vi "LINC Initialize.vi"(4 "override? registration":bool, 6 "configuration":T4={"header"=enum."STANDARD", "little endian (F)"=FALSE, "always write config (F)"=FALSE, "record commands (F)"=FALSE, "root COSMOS path (\"\")"=path "", "cmd record path (\"\")"=path "", "cmd interrupt (CMD)"="CMD", "tlm interrupt (TLM)"="TLM", "error interrupt (ERROR)"="ERROR", "default string bytes (50)"=50, "default array elements (50)"=50, "cmd length_bitoffset"=0, "cmd length_bitsize"=0, "cmd length_value_offset"=0, "tlm length_bitoffset"=0, "tlm length_bitsize"=0, "tlm length_value_offset"=0, "cmd GUID_bitoffset"=0, "tlm GUID_bitoffset"=0}, 7 "client session (F)":bool, 8 "error in (no error)":errorcluster, 9 "server name (\"\")":string, 10 "target name":string="APP", 11 "application queue":refnum<queue>) -> (0 "error out":errorcluster, 3 "LINC session":refnum<class "LINC.lvclass">)   [LabVIEW 2018, in "STEPkgDriver_LINC.lvlib" / "LINC.lvclass"]
uses:
  LINC.lvclass
  STEPkgDriver_LINC.lvlib
  LINC Global Mode.ctl
  LINC Global Session Mode.ctl
  LINC Global Config Mode.ctl
  LINC CCSDS Callback.vi
  LINC Config.ctl
  LINC Standard Callback.vi
  LINC Global Handshake Mode.ctl
  LINC Global ID Mode.ctl
  LINC Daemon Manager Mode.ctl
  LINC Default Command Header.ctl
  LINC Default Telemetry Header.ctl
panel:
  in  "standard header":T1
  in  "CCSDS telemetry header":T2={"HDR_TYPE"=0, "HDR_ID"=0, "HDR_FLAGS"=3, "HDR_COUNT"=0, "HDR_LENGTH"=0, "HDR_DAY"=0, "HDR_MSEC"=0, "HDR_USEC"=0} {"HDR_COUNT" max=16383; "HDR_FLAGS" min=3 max=3; "HDR_ID" max=2047; "HDR_TYPE" max=0}
  in  "CCSDS command header":T3={"HDR_TYPE"=2, "HDR_ID"=0, "HDR_FLAGS"=3, "HDR_COUNT"=0, "HDR_LENGTH"=0} {"HDR_COUNT" max=16383; "HDR_FLAGS" min=3 max=3; "HDR_ID" max=2047; "HDR_TYPE" min=2 max=2}
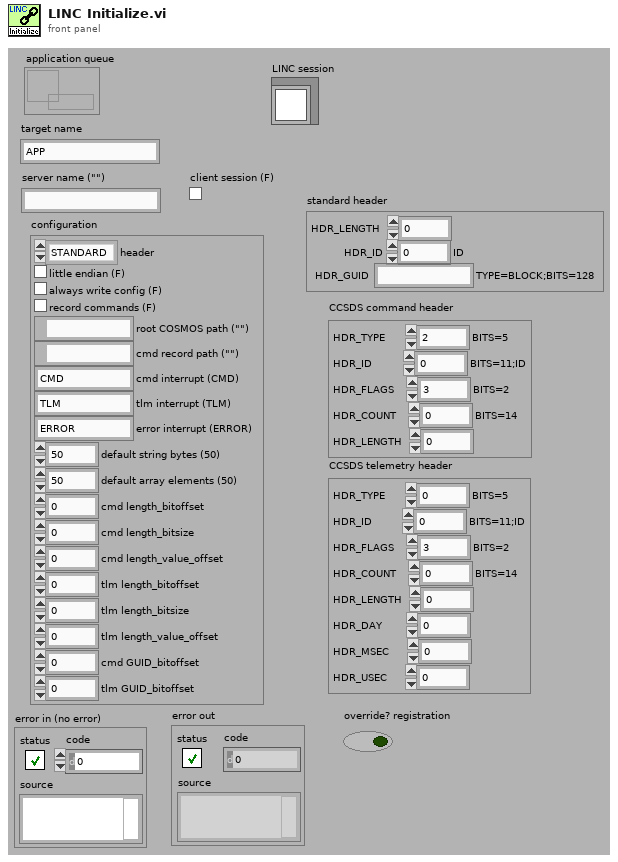
[diagram p1: front panel]
types:
  T1 = cluster{"HDR_LENGTH":u16, "HDR_ID":u16, "HDR_GUID":string}
  T2 = typedef "STEPkgDriver_LINC.lvlib/LINC Default Telemetry Header.ctl" = cluster{"HDR_TYPE":u8, "HDR_ID":u16, "HDR_FLAGS":u16, "HDR_COUNT":u16, "HDR_LENGTH":u16, "HDR_DAY":u16, "HDR_MSEC":u32, "HDR_USEC":u16}
  T3 = typedef "STEPkgDriver_LINC.lvlib/LINC Default Command Header.ctl" = cluster{"HDR_TYPE":u8, "HDR_ID":u16, "HDR_FLAGS":u16, "HDR_COUNT":u16, "HDR_LENGTH":u16}
  T4 = cluster{"header":enum16{"STANDARD", "CCSDS", "CUSTOM"}, "little endian (F)":bool, "always write config (F)":bool, "record commands (F)":bool, "root COSMOS path (\"\")":path, "cmd record path (\"\")":path, "cmd interrupt (CMD)":string, "tlm interrupt (TLM)":string, "error interrupt (ERROR)":string, "default string bytes (50)":i32, "default array elements (50)":i32, "cmd length_bitoffset":i32, "cmd length_bitsize":i32, "cmd length_value_offset":i32, "tlm length_bitoffset":i32, "tlm length_bitsize":i32, "tlm length_value_offset":i32, "cmd GUID_bitoffset":i32, "tlm GUID_bitoffset":i32}
  T5 = typedef "STEPkgDriver_LINC.lvlib/LINC Daemon Manager Mode.ctl" = enum16{"INIT", "CLEAR", "GET"}
  T6 = typedef "STEPkgDriver_LINC.lvlib/LINC Global ID Mode.ctl" = enum16{"INIT", "CLEAR", "GET_ID"}
  T7 = typedef "STEPkgDriver_LINC.lvlib/LINC Global Handshake Mode.ctl" = enum16{"INIT", "CLEAR", "ADD_COMMAND", "RMV_COMMAND", "CLR_HANDSHAKE", "SET_HANDSHAKE", "GET_HANDSHAKE"}
  T8 = typedef "STEPkgDriver_LINC.lvlib/LINC Global Session Mode.ctl" = enum16{"INIT", "CLEAR", "ADD_SESSION", "SET_CONNECTION", "SET_LISTENER", "SET_REFERENCE", "GET_SESSION"}
  T9 = typedef "STEPkgDriver_LINC.lvlib/LINC Global Config Mode.ctl" = enum16{"INIT", "CLEAR", "SET_CMD_CB", "SET_TLM_CB", "SET_CMD_FIELDS", "SET_TLM_FIELDS", "SET_ID", "GET_CONFIG"}
  T10 = typedef "STEPkgDriver_LINC.lvlib/LINC Global Mode.ctl" = enum16{"INIT", "CLEAR", "ADD_PKT_HDR", "ADD_PKT", "GET_PKT_NAMES", "GET_PKT_DESC", "GET_PKT_HDR", "GET_PKT", "SET_PKT", "SET_DATA", "SIM_EN", "SIM_DS"}
  T11 = typedef "STEPkgDriver_LINC.lvlib/LINC Config.ctl" = cluster{"cmd callback":refnum<vi>, "tlm callback":refnum<vi>, "cmd ID bitoffset":i32, "cmd ID bitsize":i32, "cmd IDs":i32[], "tlm ID bitoffset":i32, "tlm ID bitsize":i32, "tlm IDs":i32[], "cmd header fields":i32, "tlm header fields":i32, "tlm header size":i32}
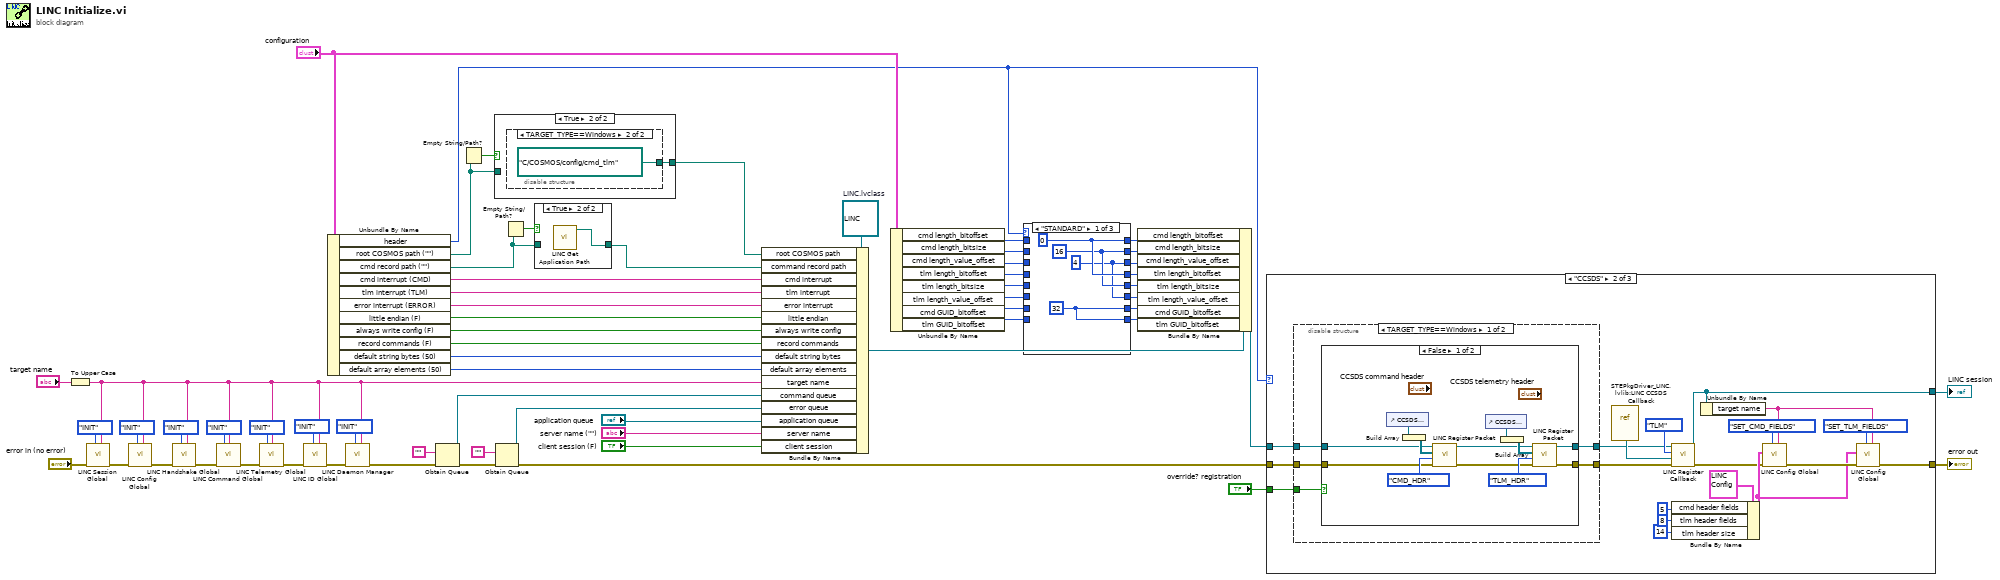
[diagram p0: block diagram]
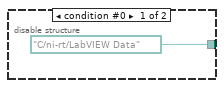
[diagram p3: hidden frame]
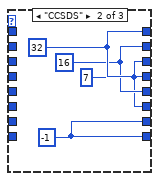
[diagram p4: hidden frame]
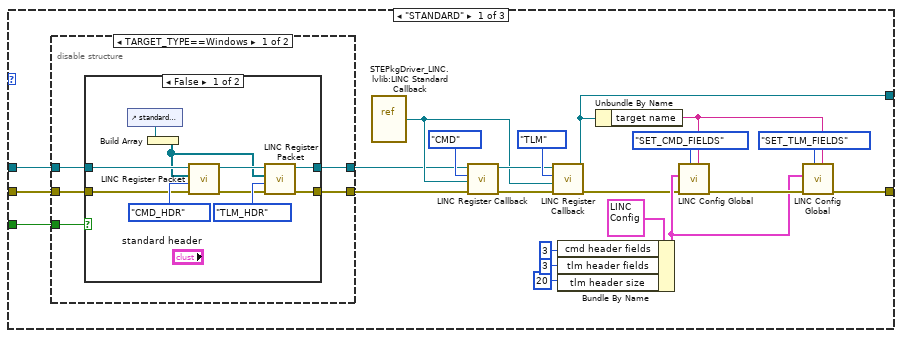
[diagram p6: hidden frame]
diagram:
  w49 = refnum<class "LINC.lvclass"> refnum  # LINC.lvclass
  n1 = To Upper Case(1:"target name") -> (0:w2:string)
  n2 = call "LINC Session Global.vi"("target name"=w2, "mode"=LINC_Global_Session_Mode."INIT", "error in (no error)"="error in (no error)") -> ("error out"=w52:errorcluster)  [unwired: 4 in, 4 out]
  n3 = call "LINC Config Global.vi"("target name"=w2, "mode"=LINC_Global_Config_Mode."INIT", "error in (no error)"=w52) -> ("error out"=w19:errorcluster)  [unwired: 7 in, 1 out]
  n4 = call "LINC Handshake Global.vi"("target name"=w2, "mode"=LINC_Global_Handshake_Mode."INIT", "error in (no error)"=w19) -> ("error out"=w18:errorcluster)  [unwired: 5 in, 3 out]
  n5 = call "LINC Command Global.vi"("mode"=LINC_Global_Mode."INIT", "target name"=w2, "error in (no error)"=w18) -> ("error out"=w63:errorcluster)  [unwired: 8 in, 4 out]
  n6 = call "LINC Telemetry Global.vi"("mode"=LINC_Global_Mode."INIT", "target name"=w2, "error in (no error)"=w63) -> ("error out"=w8:errorcluster)  [unwired: 8 in, 4 out]
  n7 = call "LINC ID Global.vi"("target name"=w2, "mode"=LINC_Global_ID_Mode."INIT", "error in (no error)"=w8) -> ("error out"=w4:errorcluster)  [unwired: 7 in, 1 out]
  n8 = Unbundle By Name("configuration") -> ("header"=w38:enum16{"STANDARD", "CCSDS", "CUSTOM"}, "root COSMOS path (\"\")"=w15:path, "cmd record path (\"\")"=w60:path, "cmd interrupt (CMD)"=w61:string, "tlm interrupt (TLM)"=w54:string, "error interrupt (ERROR)"=w13:string, "little endian (F)"=w43:bool, "always write config (F)"=w42:bool, "record commands (F)"=w41:bool, "default string bytes (50)"=w64:i32, "default array elements (50)"=w62:i32)
  n9 = call "LINC Daemon Manager.vi"("target name"=w2, "mode"=LINC_Daemon_Manager_Mode."INIT", "error in (no error)"=w4) -> ("error out"=w3:errorcluster)  [unwired: 7 in, 1 out]
  n10 = Obtain Queue(element data type="", error in (no error)=w3) -> (queue out=w48:refnum<queue>, error out=w11:errorcluster)  [unwired: 3 in, 1 out]
  n11 = Empty String/Path?(string/path=w15) -> (empty?=w16:bool)
  n12 = case shown="True" w16 {
    tunnel: w15 -> [w65 _]
    tunnel: [w65 w66] -> w14
    frame False {
    }
    frame True {
      n13 = disable-structure shown="TARGET_TYPE==Windows" {
        disable-tunnel: [path "C:/ni-rt/LabVIEW Data" ("Root COSMOS path") path "C:/COSMOS/config/cmd_tlm" ("Root COSMOS path")] -> w66
        frame condition #0 {
        }
        frame condition #1 (active) {
        }
      }
    }
  }
  n14 = Obtain Queue(element data type="", error in (no error)=w11) -> (queue out=w9:refnum<queue>, error out=w10:errorcluster)  [unwired: 3 in, 1 out]
  n15 = Empty String/Path?(string/path=w60) -> (empty?=w59:bool)
  n16 = case shown="True" w59 {
    tunnel: w60 -> [w69 _]
    tunnel: [w69 w70] -> w58
    frame False {
    }
    frame True {
      n17 = call "LINC Get Application Path.vi"() -> ("application path"=w70:path)  [unwired: 10 in, 1 out]
    }
  }
  n18 = Bundle By Name(cluster=w49, "root COSMOS path"=w14, "command record path"=w58, "cmd interrupt"=w61, "tlm interrupt"=w54, "error interrupt"=w13, "little endian"=w43, "always write config"=w42, "record commands"=w41, "default string bytes"=w64, "default array elements"=w62, "target name"=w2, "command queue"=w48, "error queue"=w9, "application queue"="application queue", "server name"="server name (\"\")", "client session"="client session (F)") -> (w37:refnum<class "LINC.lvclass">)
  n19 = Unbundle By Name("configuration") -> ("cmd length_bitoffset"=w35:i32, "cmd length_bitsize"=w28:i32, "cmd length_value_offset"=w27:i32, "tlm length_bitoffset"=w26:i32, "tlm length_bitsize"=w25:i32, "tlm length_value_offset"=w24:i32, "cmd GUID_bitoffset"=w22:i32, "tlm GUID_bitoffset"=w21:i32)
  n20 = case shown="\"STANDARD\"" w38 {
    tunnel: w35 -> [_ _ w86]
    tunnel: [w74 w78 w86] -> w34
    tunnel: [w73 w77 w85] -> w33
    tunnel: [w72 w76 w84] -> w32
    tunnel: [w74 w78 w83] -> w31
    tunnel: [w73 w77 w82] -> w30
    tunnel: [w72 w76 w81] -> w29
    tunnel: w28 -> [_ _ w85]
    tunnel: w27 -> [_ _ w84]
    tunnel: w26 -> [_ _ w83]
    tunnel: w25 -> [_ _ w82]
    tunnel: w24 -> [_ _ w81]
    tunnel: [w71 w75 w80] -> w23
    tunnel: w22 -> [_ _ w80]
    tunnel: w21 -> [_ _ w79]
    tunnel: [w71 w75 w79] -> w20
    frame "STANDARD" {
      w71 = 32
      w72 = 4
      w73 = 16
      w74 = 0
    }
    frame "CCSDS" {
      w75 = -1
      w76 = 7
      w77 = 16
      w78 = 32
    }
    frame "CUSTOM" {
    }
  }
  n21 = Bundle By Name(cluster=w37, "cmd length_bitoffset"=w34, "cmd length_bitsize"=w33, "cmd length_value_offset"=w32, "tlm length_bitoffset"=w31, "tlm length_bitsize"=w30, "tlm length_value_offset"=w29, "cmd GUID_bitoffset"=w23, "tlm GUID_bitoffset"=w20) -> (w36:refnum<class "LINC.lvclass">)
  n22 = case shown="\"CCSDS\"" w38 {
    tunnel: w10 -> [w108 w146 w169]
    tunnel: [w103 w130 w169] -> w44
    tunnel: w36 -> [w107 w145 w168]
    tunnel: [w90 w129 w168] -> w40
    tunnel: "override? registration" -> [w87 w128 _]
    frame "STANDARD" {
      n23 = disable-structure shown="TARGET_TYPE==Windows" {
        disable-tunnel: w108 -> [w113 w126]
        disable-tunnel: w107 -> [w112 w127]
        disable-tunnel: [w111 w126] -> w94
        disable-tunnel: [w110 w127] -> w89
        disable-tunnel: w87 -> [w109 _]
        frame condition #0 (active) {
          n24 = case shown="False" w109 {
            tunnel: w113 -> [w122 w125]
            tunnel: w112 -> [w119 w124]
            tunnel: [w115 w125] -> w111
            tunnel: [w114 w124] -> w110
            frame False {
              n25 = control-ref of="standard header"() -> (w117:refnum<vi>)
              n26 = Build Array(w117) -> (w116:refnum<vi>[])
              n27 = call "LINC Register Packet.vi"("error in (no error)"=w122, "type (CMD)"=enum16{"CMD", "TLM", "CMD_HDR", "TLM_HDR"}."CMD_HDR", "controls"=w116, "LINC session"=w119) -> ("error out"=w120:errorcluster, "dup LINC session"=w118:refnum<class "LINC.lvclass">)  [unwired: 6 in]
              n28 = call "LINC Register Packet.vi"("error in (no error)"=w120, "type (CMD)"=enum16{"CMD", "TLM", "CMD_HDR", "TLM_HDR"}."TLM_HDR", "controls"=w116, "LINC session"=w118) -> ("error out"=w115:errorcluster, "dup LINC session"=w114:refnum<class "LINC.lvclass">)  [unwired: 6 in]
            }
            frame True {
            }
          }
        }
        frame condition #1 {
        }
      }
      n29 = vi-ref "STEPkgDriver_LINC.lvlib:LINC Standard Callback.vi"() -> (w91:refnum<vi>)
      n30 = call "LINC Register Callback.vi"("error in (no error)"=w94, "callback ref"=w91, "mode (cmd)"=enum16{"CMD", "TLM"}."CMD", "LINC session"=w89) -> ("error out"=w93:errorcluster, "dup LINC session"=w92:refnum<class "LINC.lvclass">)  [unwired: 6 in]
      n31 = call "LINC Register Callback.vi"("error in (no error)"=w93, "callback ref"=w91, "mode (cmd)"=enum16{"CMD", "TLM"}."TLM", "LINC session"=w92) -> ("error out"=w88:errorcluster, "dup LINC session"=w90:refnum<class "LINC.lvclass">)  [unwired: 6 in]
      n32 = Bundle By Name(cluster=T11 {"cmd callback"=refnum, "tlm callback"=refnum, "cmd ID bitoffset"=0, "cmd ID bitsize"=0, "cmd IDs"=[], "tlm ID bitoffset"=0, "tlm ID bitsize"=0, "tlm IDs"=[], "cmd header fields"=0, "tlm header fields"=0, "tlm header size"=0} ("config in"), "cmd header fields"=3, "tlm header fields"=3, "tlm header size"=20) -> (w100:T11)
      n33 = Unbundle By Name(w90) -> ("target name"=w102:string)
      n34 = call "LINC Config Global.vi"("target name"=w102, "mode"=LINC_Global_Config_Mode."SET_CMD_FIELDS", "error in (no error)"=w88, "config in"=w100) -> ("error out"=w104:errorcluster)  [unwired: 6 in, 1 out]
      n35 = call "LINC Config Global.vi"("target name"=w102, "mode"=LINC_Global_Config_Mode."SET_TLM_FIELDS", "error in (no error)"=w104, "config in"=w100) -> ("error out"=w103:errorcluster)  [unwired: 6 in, 1 out]
    }
    frame "CCSDS" {
      n36 = disable-structure shown="TARGET_TYPE==Windows" {
        disable-tunnel: w146 -> [w151 w166]
        disable-tunnel: w145 -> [w150 w167]
        disable-tunnel: [w149 w166] -> w142
        disable-tunnel: [w148 w167] -> w141
        disable-tunnel: w128 -> [w147 _]
        frame condition #0 (active) {
          n37 = case shown="False" w147 {
            tunnel: w151 -> [w160 w164]
            tunnel: w150 -> [w155 w165]
            tunnel: [w153 w164] -> w149
            tunnel: [w152 w165] -> w148
            frame False {
              n38 = control-ref of="CCSDS command header"() -> (w161:refnum<vi>)
              n39 = Build Array(w161) -> (w163:refnum<vi>[])
              n40 = call "LINC Register Packet.vi"("error in (no error)"=w160, "type (CMD)"=enum16{"CMD", "TLM", "CMD_HDR", "TLM_HDR"}."CMD_HDR", "controls"=w163, "LINC session"=w155) -> ("error out"=w156:errorcluster, "dup LINC session"=w154:refnum<class "LINC.lvclass">)  [unwired: 6 in]
              n41 = control-ref of="CCSDS telemetry header"() -> (w157:refnum<vi>)
              n42 = Build Array(w157) -> (w159:refnum<vi>[])
              n43 = call "LINC Register Packet.vi"("error in (no error)"=w156, "type (CMD)"=enum16{"CMD", "TLM", "CMD_HDR", "TLM_HDR"}."TLM_HDR", "controls"=w159, "LINC session"=w154) -> ("error out"=w153:errorcluster, "dup LINC session"=w152:refnum<class "LINC.lvclass">)  [unwired: 6 in]
            }
            frame True {
            }
          }
        }
        frame condition #1 {
        }
      }
      n44 = vi-ref "STEPkgDriver_LINC.lvlib:LINC CCSDS Callback.vi"() -> (w143:refnum<vi>)
      n45 = call "LINC Register Callback.vi"("error in (no error)"=w142, "callback ref"=w143, "mode (cmd)"=enum16{"CMD", "TLM"}."TLM", "LINC session"=w141) -> ("error out"=w131:errorcluster, "dup LINC session"=w129:refnum<class "LINC.lvclass">)  [unwired: 6 in]
      n46 = Bundle By Name(cluster=T11 {"cmd callback"=refnum, "tlm callback"=refnum, "cmd ID bitoffset"=0, "cmd ID bitsize"=0, "cmd IDs"=[], "tlm ID bitoffset"=0, "tlm ID bitsize"=0, "tlm IDs"=[], "cmd header fields"=0, "tlm header fields"=0, "tlm header size"=0} ("config in"), "cmd header fields"=5, "tlm header fields"=8, "tlm header size"=14) -> (w135:T11)
      n47 = Unbundle By Name(w129) -> ("target name"=w137:string)
      n48 = call "LINC Config Global.vi"("target name"=w137, "mode"=LINC_Global_Config_Mode."SET_CMD_FIELDS", "error in (no error)"=w131, "config in"=w135) -> ("error out"=w138:errorcluster)  [unwired: 6 in, 1 out]
      n49 = call "LINC Config Global.vi"("target name"=w137, "mode"=LINC_Global_Config_Mode."SET_TLM_FIELDS", "error in (no error)"=w138, "config in"=w135) -> ("error out"=w130:errorcluster)  [unwired: 6 in, 1 out]
    }
    frame "CUSTOM" {
    }
  }
  "error out" <- w44
  "LINC session" <- w40
